vi "Set Pump Parameters (SubVI).vi"(0 "Units":string, 1 "error out 2":errorcluster, 2 "Target Volume":dbl, 5 "Flow rate":dbl, 6 "Direction":string(combo), 7 "Pump Add":string, 8 "diameter (mm)":dbl, 9 "Send":bool, 10 "VISA resource name out 2":refnum<visa-resource-name>) -> (3 "VISA resource name out":refnum<visa-resource-name>, 4 "error out":errorcluster)   [LabVIEW 2020]
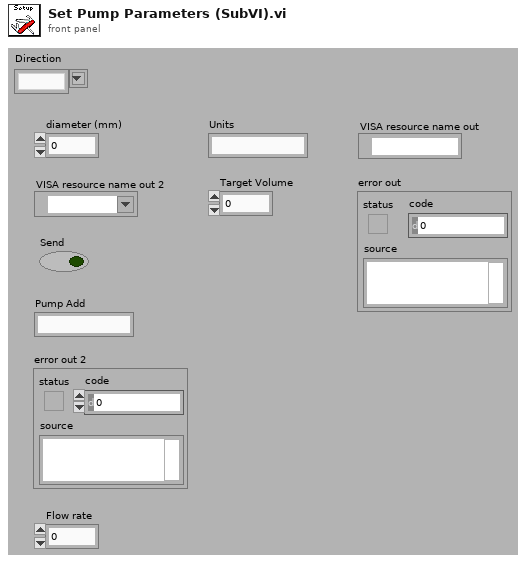
[diagram p1: front panel]
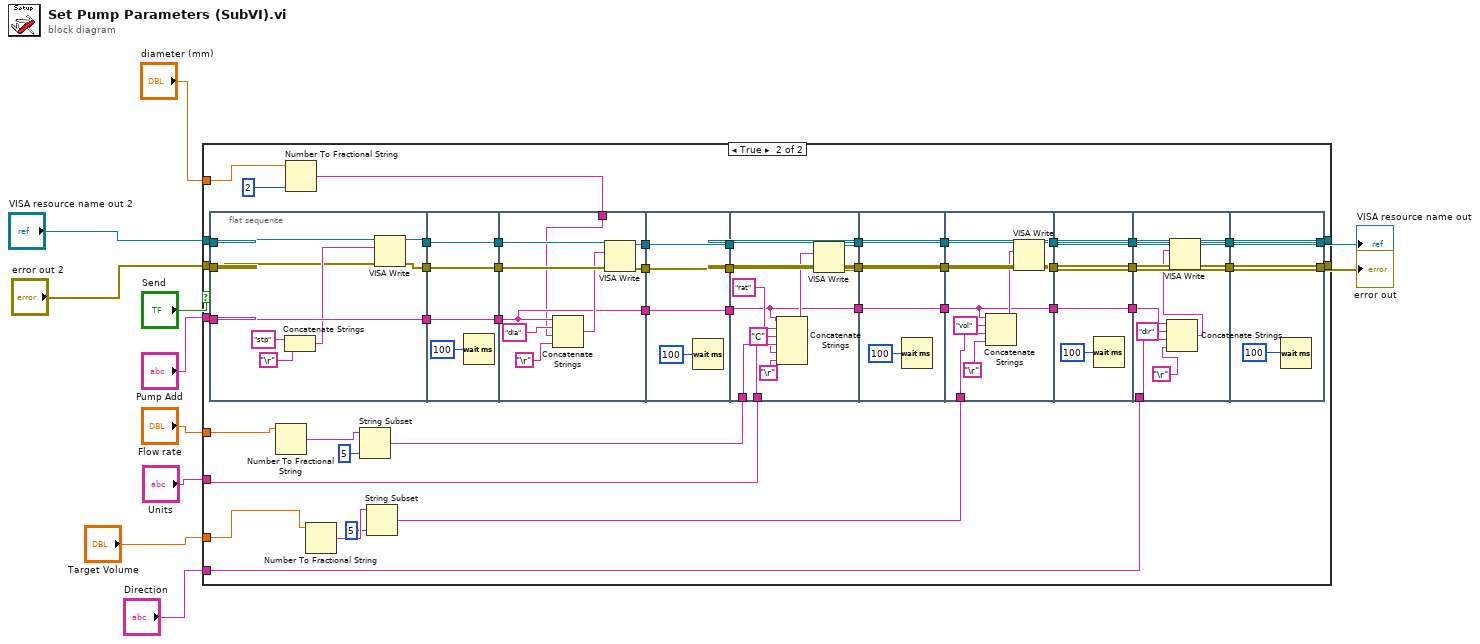
[diagram p0: block diagram]
diagram:
  n1 = case shown="True" "Send" {
    tunnel: "VISA resource name out 2" -> [w13 w57]
    tunnel: "error out 2" -> [w12 w56]
    tunnel: [w13 w55] -> w10
    tunnel: [w12 w54] -> w11
    tunnel: "Pump Add" -> [_ w53]
    tunnel: "diameter (mm)" -> [_ w23]
    tunnel: "Flow rate" -> [_ w24]
    tunnel: "Units" -> [_ w52]
    tunnel: "Target Volume" -> [_ w20]
    tunnel: "Direction" -> [_ w33]
    frame False {
    }
    frame True {
      n2 = flat-sequence {
        tunnel: w53 -> [w65]
        tunnel: w56 -> [w60]
        tunnel: w57 -> [w61]
        tunnel: [w59] -> w19
        tunnel: [w58] -> w17
        tunnel: [w65] -> w15
        tunnel: w19 -> [w69]
        tunnel: [w69] -> w18
        tunnel: w17 -> [w68]
        tunnel: [w68] -> w16
        tunnel: w15 -> [w67]
        tunnel: [w67] -> w14
        tunnel: [w76] -> w51
        tunnel: [w75] -> w49
        tunnel: [w71] -> w47
        tunnel: w22 -> [w70]
        tunnel: w18 -> [w78]
        tunnel: w16 -> [w77]
        tunnel: w14 -> [w71]
        tunnel: w51 -> [w82]
        tunnel: [w82] -> w50
        tunnel: w49 -> [w81]
        tunnel: [w81] -> w48
        tunnel: w47 -> [w80]
        tunnel: [w80] -> w46
        tunnel: w50 -> [w93]
        tunnel: w48 -> [w91]
        tunnel: w46 -> [w84]
        tunnel: w29 -> [w88]
        tunnel: w52 -> [w87]
        tunnel: [w92] -> w45
        tunnel: [w90] -> w43
        tunnel: [w84] -> w41
        tunnel: w45 -> [w97]
        tunnel: [w97] -> w44
        tunnel: w43 -> [w96]
        tunnel: [w96] -> w42
        tunnel: w41 -> [w95]
        tunnel: [w95] -> w40
        tunnel: w44 -> [w104]
        tunnel: w42 -> [w103]
        tunnel: w40 -> [w98]
        tunnel: w25 -> [w100]
        tunnel: [w105] -> w39
        tunnel: [w106] -> w38
        tunnel: [w98] -> w35
        tunnel: w39 -> [w110]
        tunnel: w38 -> [w109]
        tunnel: [w110] -> w37
        tunnel: [w109] -> w36
        tunnel: w35 -> [w107]
        tunnel: [w107] -> w34
        tunnel: w37 -> [w119]
        tunnel: w36 -> [w116]
        tunnel: w34 -> [w113]
        tunnel: w33 -> [w111]
        tunnel: [w118] -> w32
        tunnel: [w117] -> w31
        tunnel: [w121] -> w54
        tunnel: [w122] -> w55
        tunnel: w32 -> [w122]
        tunnel: w31 -> [w121]
        frame #0 {
          n3 = Concatenate Strings("stp" ("string"), "\r") -> (w62:string)
          n4 = VISA Write(VISA resource name=w61, write buffer=w62, error in (no error)=w60) -> (VISA resource name out=w59:refnum<visa-resource-name>, error out=w58:errorcluster)  [unwired: 1 out]
        }
        frame #1 {
          n5 = Wait (ms)(milliseconds to wait=u32 100) -> ()  [unwired: 1 out]
        }
        frame #2 {
          n6 = Concatenate Strings(w71, "dia" ("string"), w70, "\r") -> (w73:string)
          n7 = VISA Write(VISA resource name=w78, write buffer=w73, error in (no error)=w77) -> (VISA resource name out=w76:refnum<visa-resource-name>, error out=w75:errorcluster)  [unwired: 1 out]
        }
        frame #3 {
          n8 = Wait (ms)(milliseconds to wait=u32 100) -> ()  [unwired: 1 out]
        }
        frame #4 {
          n9 = Concatenate Strings(w84, "rat" ("string"), "C" ("string"), w88, w87, "\r") -> (w85:string)
          n10 = VISA Write(VISA resource name=w93, write buffer=w85, error in (no error)=w91) -> (VISA resource name out=w92:refnum<visa-resource-name>, error out=w90:errorcluster)  [unwired: 1 out]
        }
        frame #5 {
          n11 = Wait (ms)(milliseconds to wait=u32 100) -> ()  [unwired: 1 out]
        }
        frame #6 {
          n12 = Concatenate Strings(w98, "vol" ("string"), w100, "\r") -> (w99:string)
          n13 = VISA Write(VISA resource name=w104, write buffer=w99, error in (no error)=w103) -> (VISA resource name out=w105:refnum<visa-resource-name>, error out=w106:errorcluster)  [unwired: 1 out]
        }
        frame #7 {
          n14 = Wait (ms)(milliseconds to wait=u32 100) -> ()  [unwired: 1 out]
        }
        frame #8 {
          n15 = Concatenate Strings(w113, "dir" ("string"), w111, "\r") -> (w115:string)
          n16 = VISA Write(VISA resource name=w119, write buffer=w115, error in (no error)=w116) -> (VISA resource name out=w118:refnum<visa-resource-name>, error out=w117:errorcluster)  [unwired: 1 out]
        }
        frame #9 {
          n17 = Wait (ms)(milliseconds to wait=u32 100) -> ()  [unwired: 1 out]
        }
      }
      n18 = Number To Fractional String(number=w24) -> (F-format string=w28:string)  [unwired: 3 in]
      n19 = Number To Fractional String(number=w23, precision (6)=2) -> (F-format string=w22:string)  [unwired: 2 in]
      n20 = Number To Fractional String(number=w20) -> (F-format string=w27:string)  [unwired: 3 in]
      n21 = String Subset(string=w28, length (rest)=5 ("length (rest)")) -> (substring=w29:string)  [unwired: 1 in]
      n22 = String Subset(string=w27, length (rest)=5 ("length (rest)")) -> (substring=w25:string)  [unwired: 1 in]
    }
  }
  "error out" <- w11
  "VISA resource name out" <- w10
